vi "Build.vi"(6 "Build Events":T1, 8 "error in (no error)":errorcluster, 11 "BuildManager in":refnum<class "BuildManager.lvclass">) -> (0 "error out":errorcluster, 3 "BuildManager out":refnum<class "BuildManager.lvclass">)   [LabVIEW 2019, in "SolutionBuilder.lvlib" / "BuildManager.lvclass"]
uses:
  BuildManager.lvclass
  BuildManager.lvclass/BuildManager.ctl
  ProjectItem/ProjectItem.lvclass
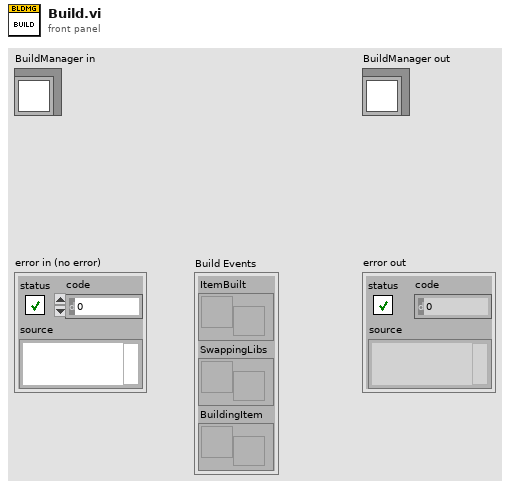
[diagram p1: front panel]
types:
  T1 = cluster{"ItemBuilt":refnum<user-event>, "SwappingLibs":refnum<user-event>, "BuildingItem":refnum<user-event>}
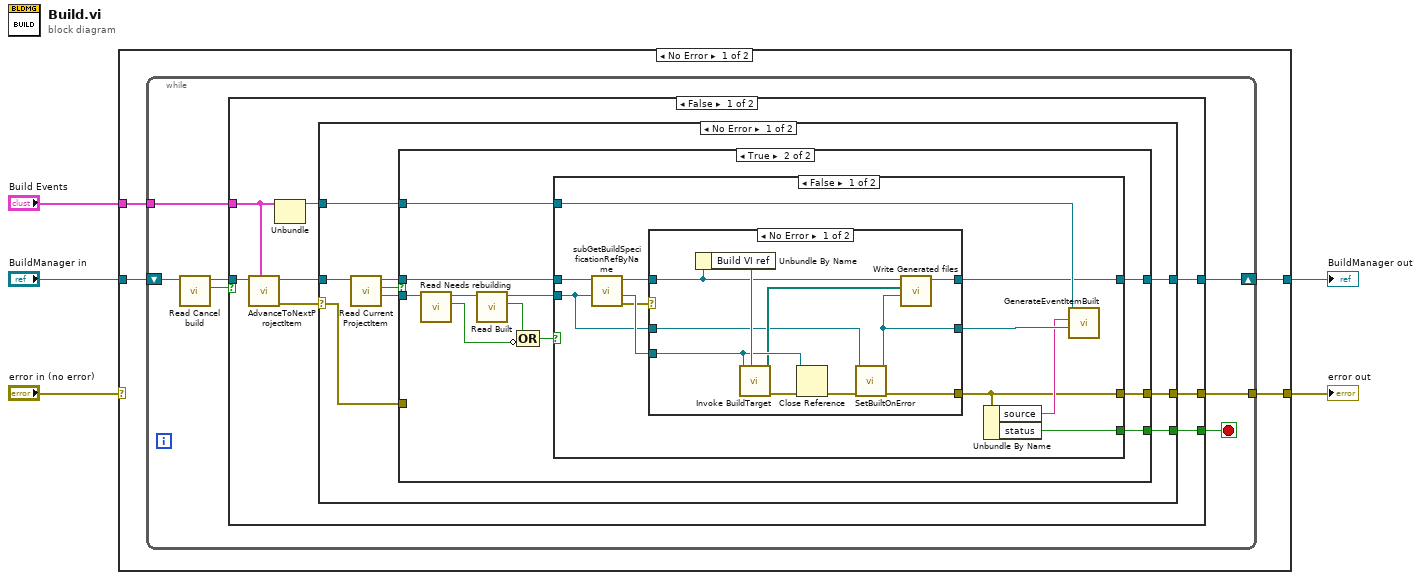
[diagram p0: block diagram]
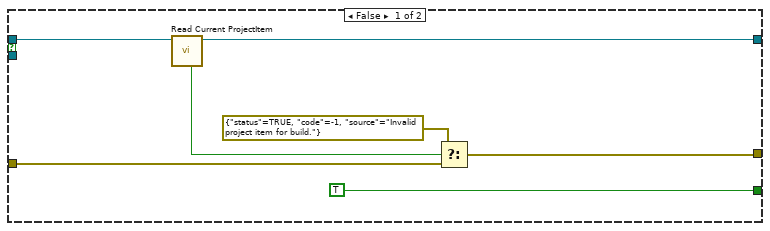
[diagram p2: hidden frame]
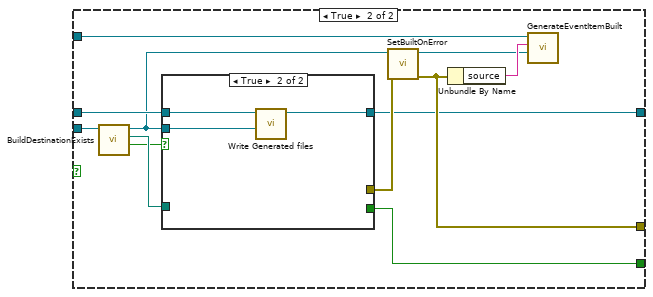
[diagram p4: hidden frame]
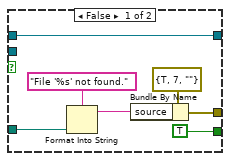
[diagram p5: hidden frame]
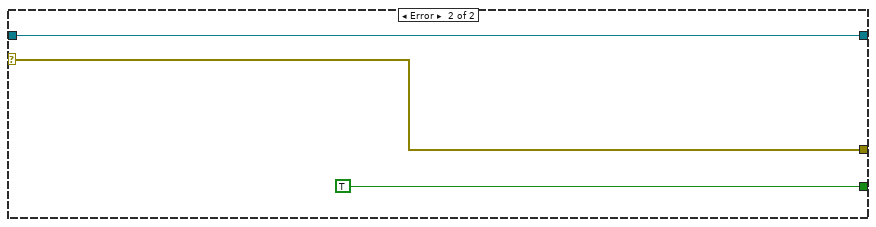
[diagram p6: hidden frame]
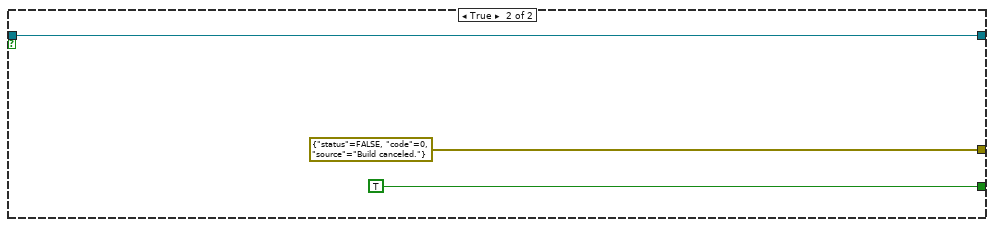
[diagram p7: hidden frame]
diagram:
  n1 = case shown="No Error" "error in (no error)" {
    selector: "error in (no error)" -> [_ w105]
    tunnel: "BuildManager in" -> [w9 w104]
    tunnel: "Build Events" -> [w8 _]
    tunnel: [w6 w105] -> w2
    tunnel: [w7 w104] -> w1
    frame No Error {
      n2 = while {
        shift-right: [w16] -> w7
        shift-left: w9 -> [w12]
        tunnel: w8 -> [w14]
        tunnel: [w13] -> w6
        stop <- w15 stop-if-true
        n3 = call "Read Cancel build.vi"("BuildManager in"=w12) -> ("Cancel?"=w10:bool, "BuildManager out"=w11:refnum<class "BuildManager.lvclass">)  [unwired: 9 in]
        n4 = case shown="False" w10 {
          tunnel: [w23 w103] -> w16
          tunnel: [w22 TRUE] -> w15
          tunnel: w14 -> [w17 _]
          tunnel: [w21 errorcluster {"status"=FALSE, "code"=0, "source"="Build canceled."} ("t")] -> w13
          tunnel: w11 -> [w19 w103]
          frame False {
            n5 = call "AdvanceToNextProjectItem.vi"("Build Events"=w17, "BuildManager in"=w19) -> ("error out"=w20:errorcluster, "BuildManager out"=w24:refnum<class "BuildManager.lvclass">)  [unwired: 8 in]
            n6 = Unbundle(w17) -> ("ItemBuilt"=w18:refnum<user-event>)  [unwired: 2 out]
            n7 = case shown="No Error" w20 {
              selector: w20 -> [w25 w98]
              tunnel: w24 -> [w33 w100]
              tunnel: [w29 w100] -> w23
              tunnel: [w28 TRUE ("status")] -> w22
              tunnel: w18 -> [w27 _]
              tunnel: [w26 w98] -> w21
              frame No Error {
                n8 = call "Read Current ProjectItem.vi"("BuildManager in"=w33) -> ("Current ProjectItem"=w30:refnum<class "ProjectItem.lvclass">, "Valid"=w32:bool, "BuildManager out"=w31:refnum<class "BuildManager.lvclass">)  [unwired: 7 in, 1 out]
                n9 = case shown="True" w32 {
                  tunnel: w31 -> [w38 w51]
                  tunnel: w30 -> [_ w44]
                  tunnel: [w39 w50] -> w29
                  tunnel: [TRUE w47] -> w28
                  tunnel: w27 -> [_ w48]
                  tunnel: [w34 w46] -> w26
                  tunnel: w25 -> [w35 _]
                  frame False {
                    n10 = call "Read Current ProjectItem.vi"("BuildManager in"=w38) -> ("BuildManager out"=w39:refnum<class "BuildManager.lvclass">, "In bounds"=w37:bool)  [unwired: 7 in, 2 out]
                    n11 = Select(t=errorcluster {"status"=TRUE, "code"=-1, "source"="Invalid project item for build."}, s=w37, f=w35) -> (s? t:f=w34:errorcluster)
                  }
                  frame True {
                    n12 = call "Read Needs rebuilding.vi"("ProjectItem in"=w44) -> ("Needs rebuilding"=w42:bool, "ProjectItem out"=w45:refnum<class "ProjectItem.lvclass">)  [unwired: 9 in]
                    n13 = call "Read Built.vi"("ProjectItem in"=w45) -> ("Built"=w43:bool, "ProjectItem out"=w49:refnum<class "ProjectItem.lvclass">)  [unwired: 9 in]
                    n14 = Compound Arithmetic op=OR(w43, invert w42) -> (w41:bool)
                    n15 = case shown="False" w41 {
                      tunnel: w51 -> [w62 w81]
                      tunnel: [w55 w80] -> w50
                      tunnel: w49 -> [w52 w79]
                      tunnel: w48 -> [w59 w84]
                      tunnel: [w57 w87] -> w47
                      tunnel: [w53 w85] -> w46
                      frame False {
                        n16 = call "subGetBuildSpecificationRefByName.vi"("ProjectItem in"=w52, "BuildManager in"=w62) -> ("error out"=w54:errorcluster, "Build spec ref"=w61:refnum<vi>, "BuildManager out"=w56:refnum<class "BuildManager.lvclass">)  [unwired: 7 in]
                        n17 = case shown="No Error" w54 {
                          selector: w54 -> [_ w73]
                          tunnel: w61 -> [w70 _]
                          tunnel: w52 -> [w64 w74]
                          tunnel: [w63 w74] -> w60
                          tunnel: [w71 w73] -> w53
                          tunnel: w56 -> [w66 w75]
                          tunnel: [w67 w75] -> w55
                          frame No Error {
                            n18 = Unbundle By Name(w66) -> ("Build VI ref"=w72:refnum<vi>)
                            n19 = call <vilib>:"Invoke BuildTarget.vi"("vi reference"=w72, "BuildItem ref"=w70) -> ("error out"=w69:errorcluster, "Generated files"=w65:path[])  [unwired: 8 in]
                            n20 = Close Reference(reference=w70, error in (no error)=w69) -> (error out=w68:errorcluster)
                            n21 = call "SetBuiltOnError.vi"("error in (no error)"=w68, "ProjectItem in"=w64) -> ("error out"=w71:errorcluster, "ProjectItem out"=w63:refnum<class "ProjectItem.lvclass">)  [unwired: 8 in]
                            n22 = call "Write Generated files.vi"("ProjectItem in"=w63, "Generated files"=w65, "BuildManager in"=w66) -> ("BuildManager out"=w67:refnum<class "BuildManager.lvclass">)  [unwired: 8 in]
                          }
                          frame Error {
                          }
                        }
                        n23 = Unbundle By Name(w53) -> ("source"=w58:string, "status"=w57:bool)
                        n24 = call "GenerateEventItemBuilt.vi"("ProjectItem"=w60, "Result"=w58, "ItemBuilt"=w59) -> ()  [unwired: 9 in]
                      }
                      frame True {
                        n25 = call "BuildDestinationExists.vi"("ProjectItem in"=w79) -> ("Exists"=w76:bool, "path out"=w77:path, "ProjectItem out"=w78:refnum<class "ProjectItem.lvclass">)  [unwired: 7 in, 1 out]
                        n26 = case shown="True" w76 {
                          tunnel: [w91 _] -> w86
                          tunnel: w77 -> [w90 _]
                          tunnel: [TRUE _] -> w87
                          tunnel: w81 -> [w88 w97]
                          tunnel: [w88 w96] -> w80
                          tunnel: w78 -> [_ w95]
                          frame False {
                            n27 = Format Into String(format string="File '%s' not found.", w90) -> (resulting string=w92:string)  [unwired: 2 in, 1 out]
                            n28 = Bundle By Name(cluster=errorcluster {"status"=TRUE, "code"=7, "source"=""} ("error out"), "source"=w92) -> (w91:errorcluster)
                          }
                          frame True {
                            n29 = call "Write Generated files.vi"("ProjectItem in"=w95, "BuildManager in"=w97) -> ("BuildManager out"=w96:refnum<class "BuildManager.lvclass">)  [unwired: 9 in]
                          }
                        }
                        n30 = call "SetBuiltOnError.vi"("error in (no error)"=w86, "ProjectItem in"=w78) -> ("error out"=w85:errorcluster, "ProjectItem out"=w82:refnum<class "ProjectItem.lvclass">)  [unwired: 8 in]
                        n31 = Unbundle By Name(w85) -> ("source"=w83:string)
                        n32 = call "GenerateEventItemBuilt.vi"("ProjectItem"=w82, "Result"=w83, "ItemBuilt"=w84) -> ()  [unwired: 9 in]
                      }
                    }
                  }
                }
              }
              frame Error {
              }
            }
          }
          frame True {
          }
        }
      }
    }
    frame Error {
    }
  }
  "error out" <- w2
  "BuildManager out" <- w1
